vi "ATM front end.vi"() -> ()   [LabVIEW 2020]
uses:
  states_enum.ctl
  <vilib>/regexp/Match Regular Expression.xnode
panel:
  out "Card LED":bool
  in  "Right Button 3":bool
  in  "Right Button 2":bool
  in  "Right Button 1":bool
  in  "Left Button 3":bool
  in  "Left Button 2":bool
  in  "Left Button 1":bool
  out "Right 3":string
  out "Right 2":string
  out "Right 1":string
  out "Left 3":string
  out "Left 2":string
  out "Left 1":string
  out "Terminal":string
  in  "User Input":string
  in  "Enter":bool
  in  "Card Simulator":bool
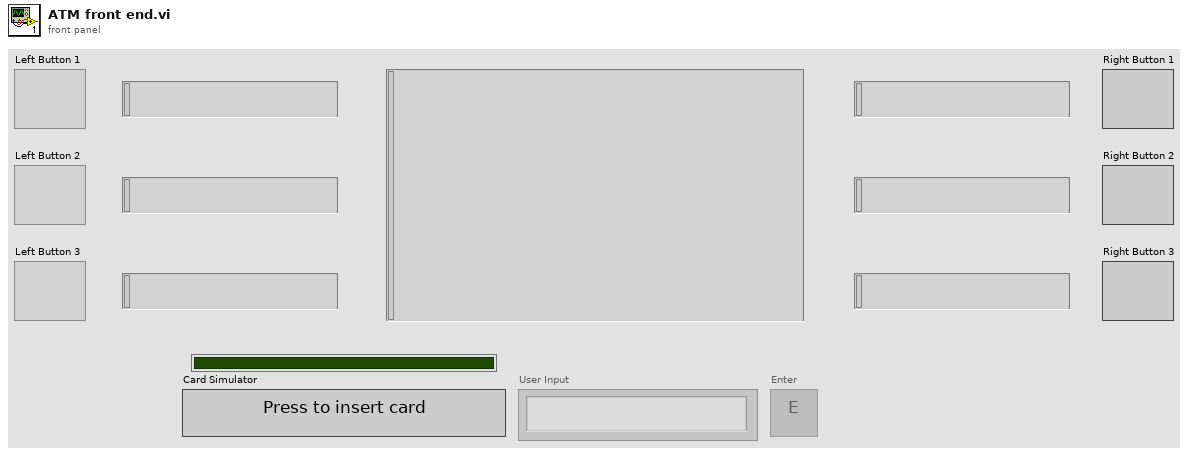
[diagram p1: front panel]
types:
  T1 = typedef "states_enum.ctl" = enum16{"Start", "Idle", "Validate card", "Enter account number", "Validate account", "Terminate session", "Main menu", "Balance Inquiry", "Deposit", "Fast Cash", "Withdraw", "Update account", "Transaction status"}
  T2 = enum8{"Enabled", "Disabled", "Disabled and Grayed Out"}
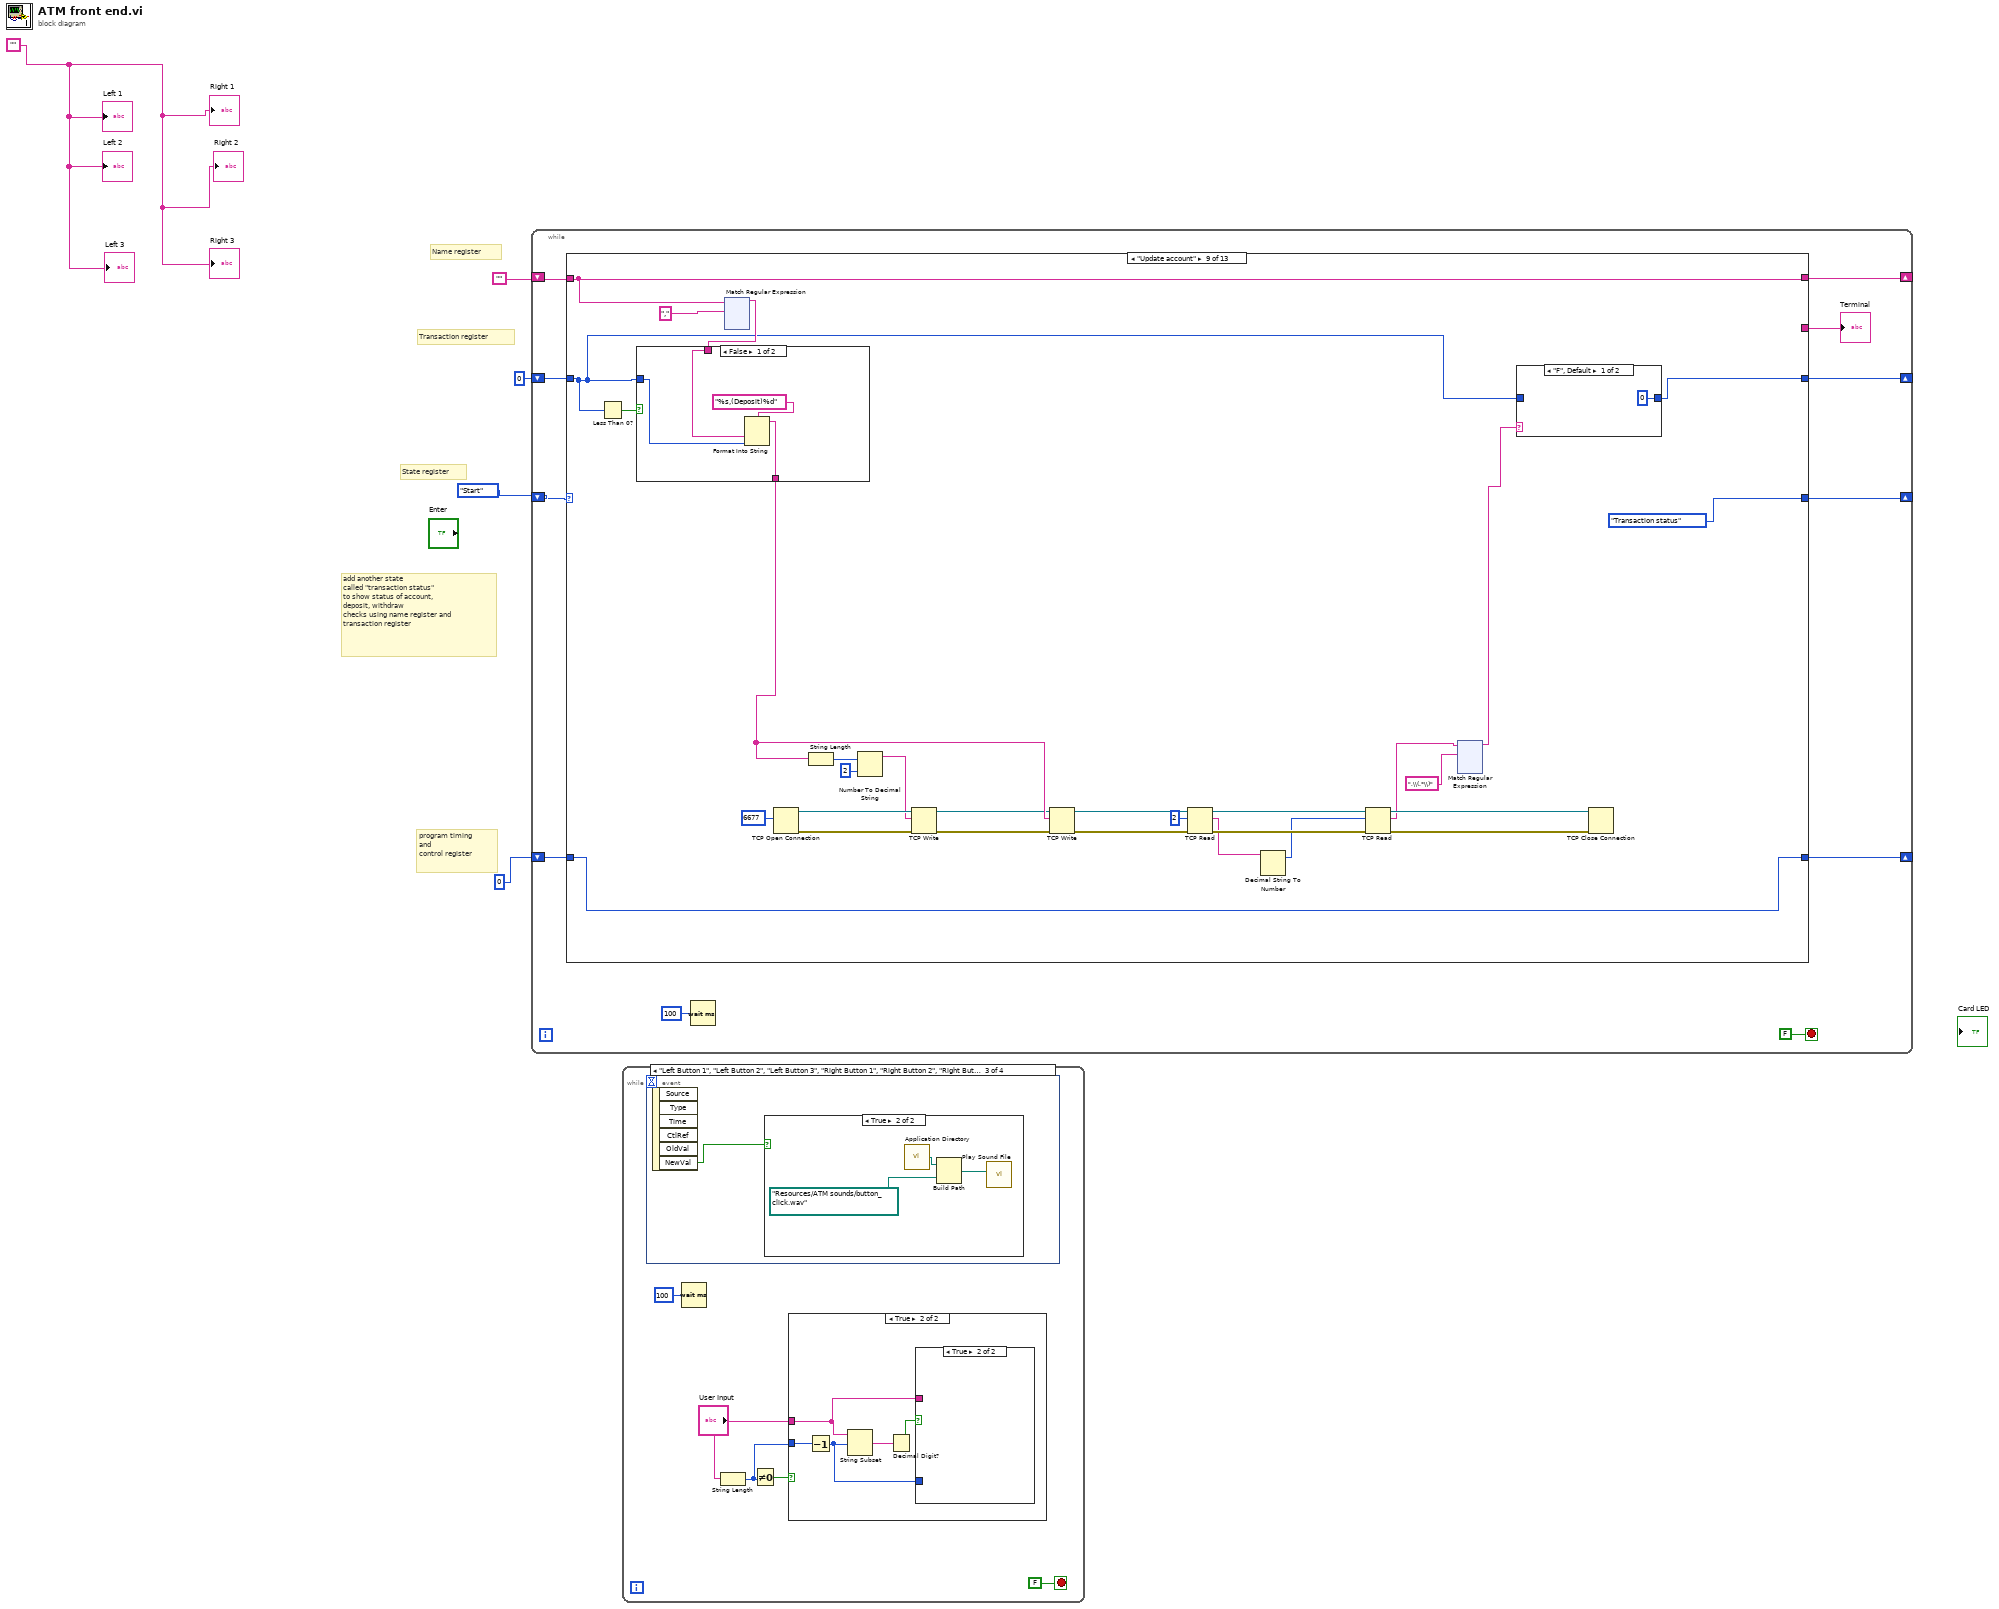
[diagram p0: block diagram]
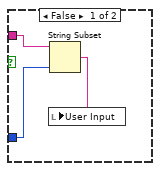
[diagram p3: hidden frame]
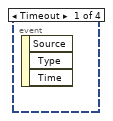
[diagram p4: hidden frame]
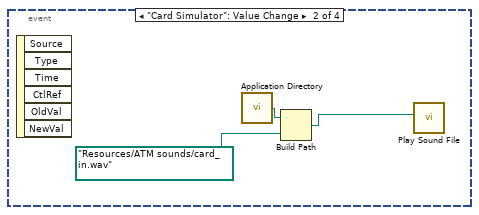
[diagram p5: hidden frame]
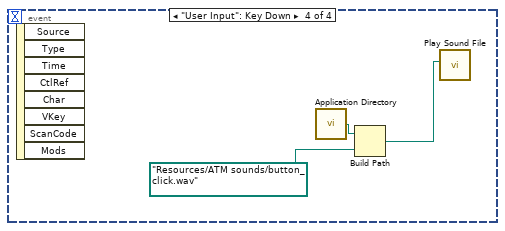
[diagram p7: hidden frame]
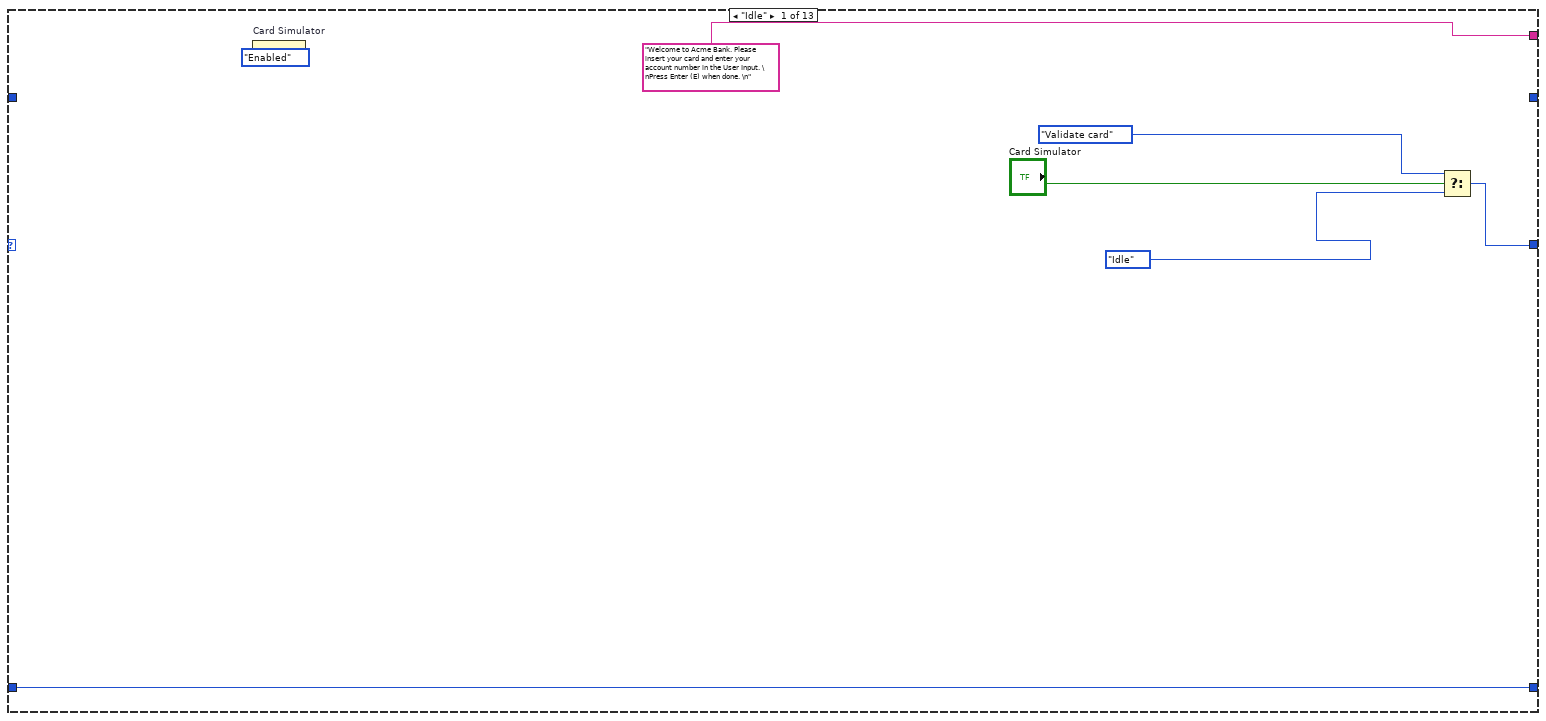
[diagram p8: hidden frame]
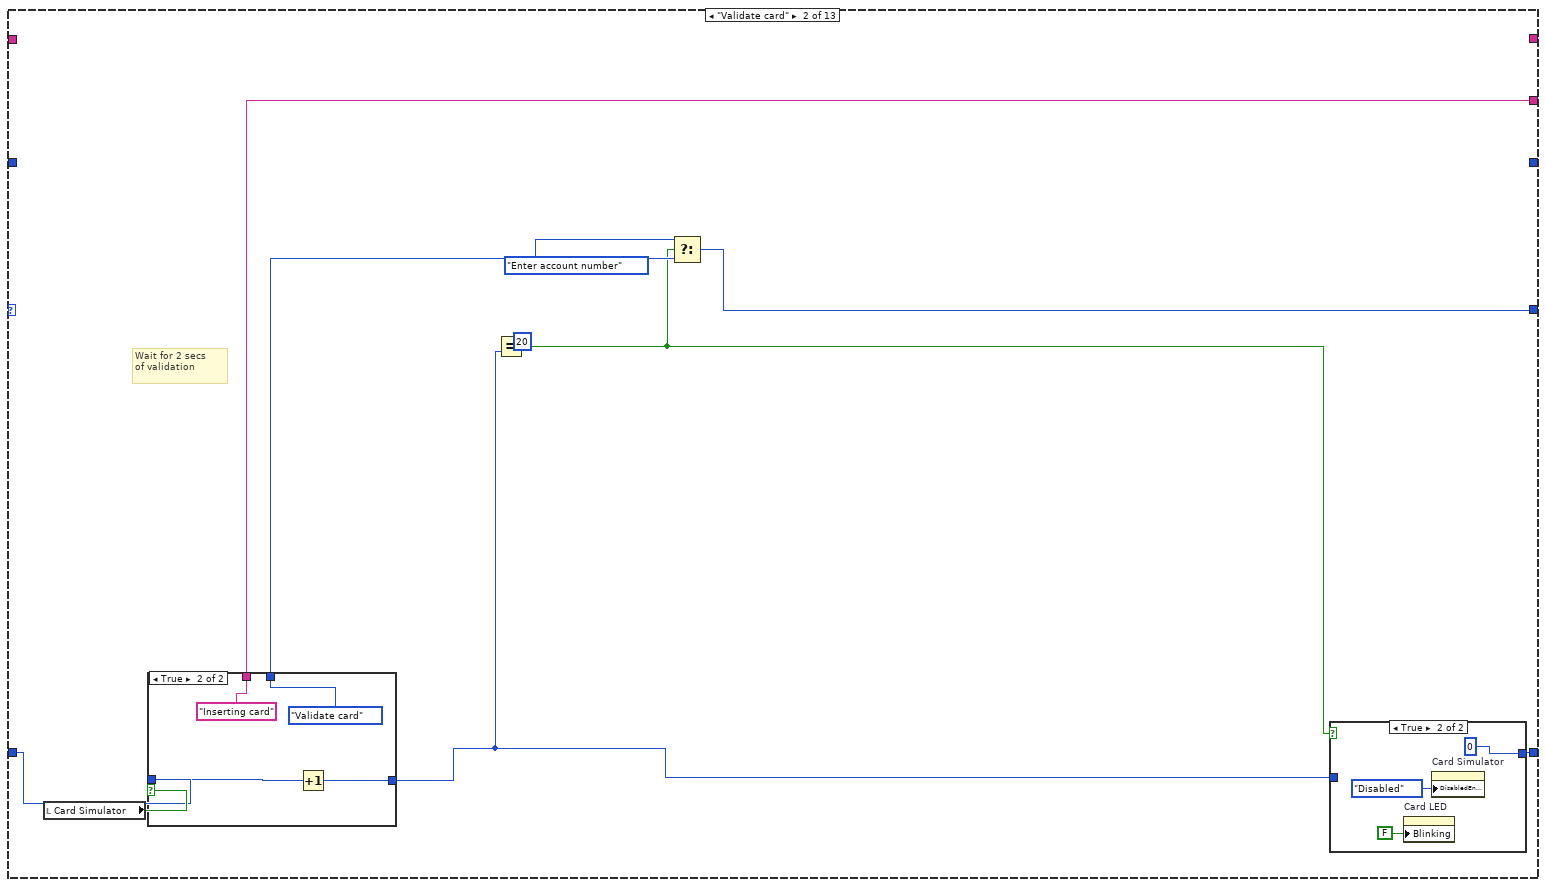
[diagram p9: hidden frame]
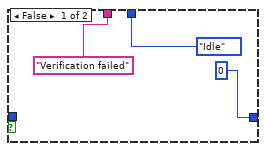
[diagram p10: hidden frame]
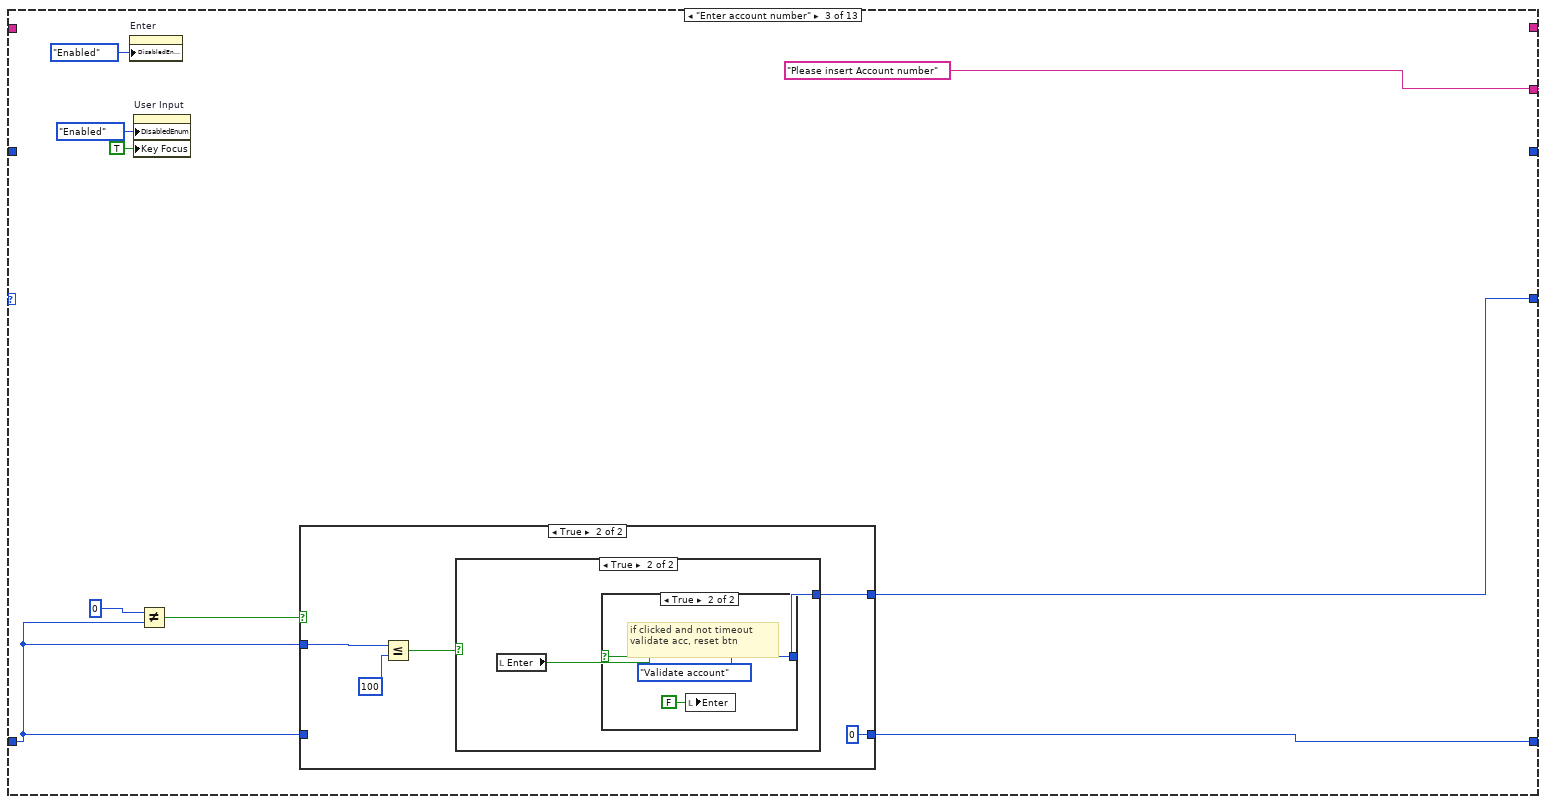
[diagram p12: hidden frame]
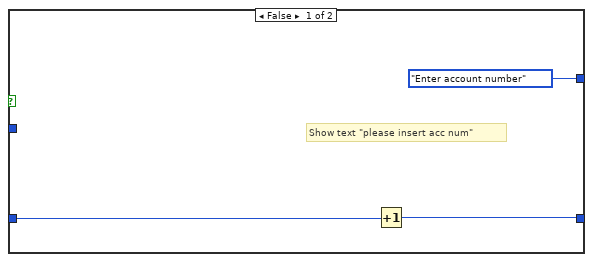
[diagram p13: hidden frame]
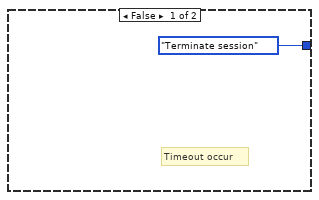
[diagram p14: hidden frame]
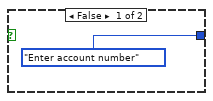
[diagram p15: hidden frame]
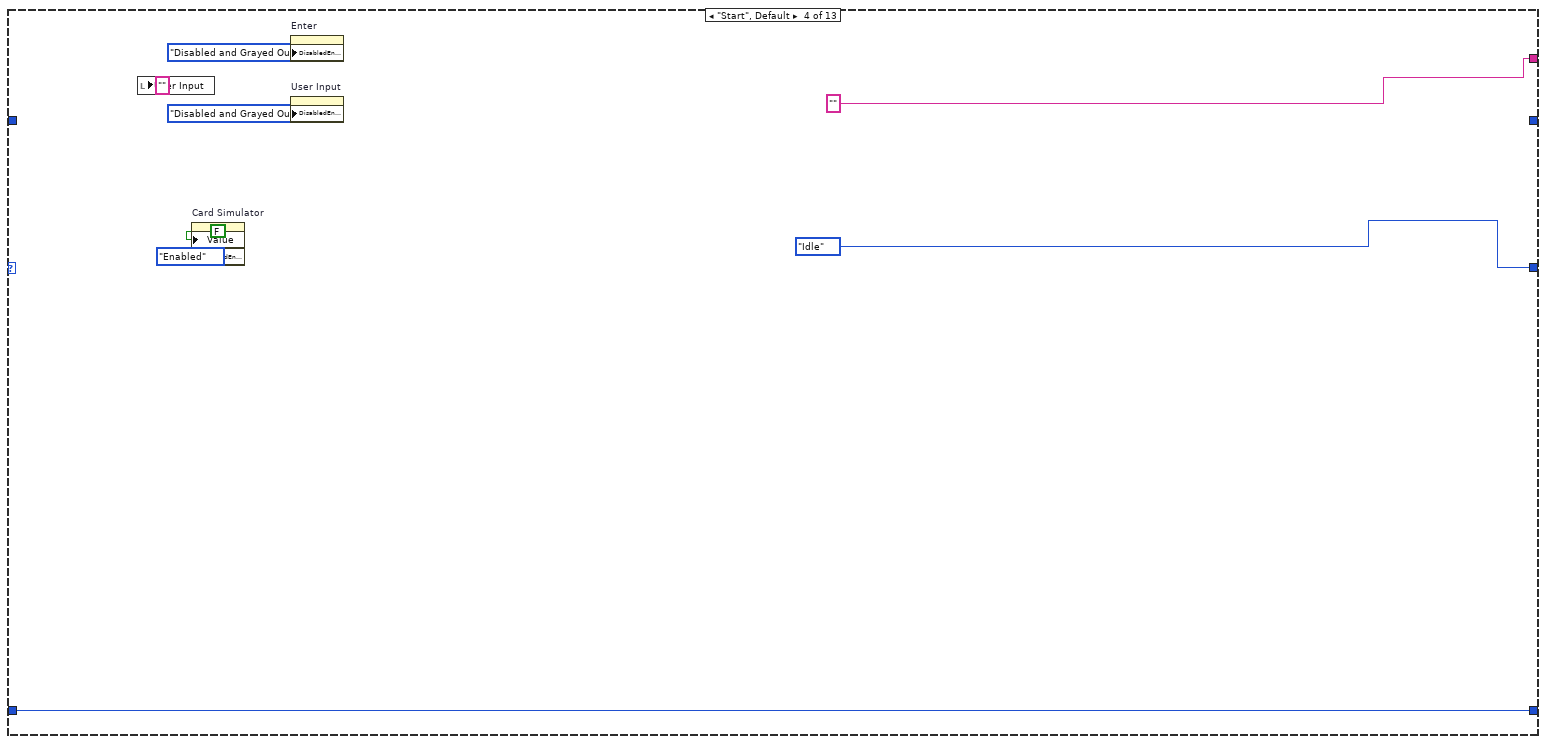
[diagram p16: hidden frame]
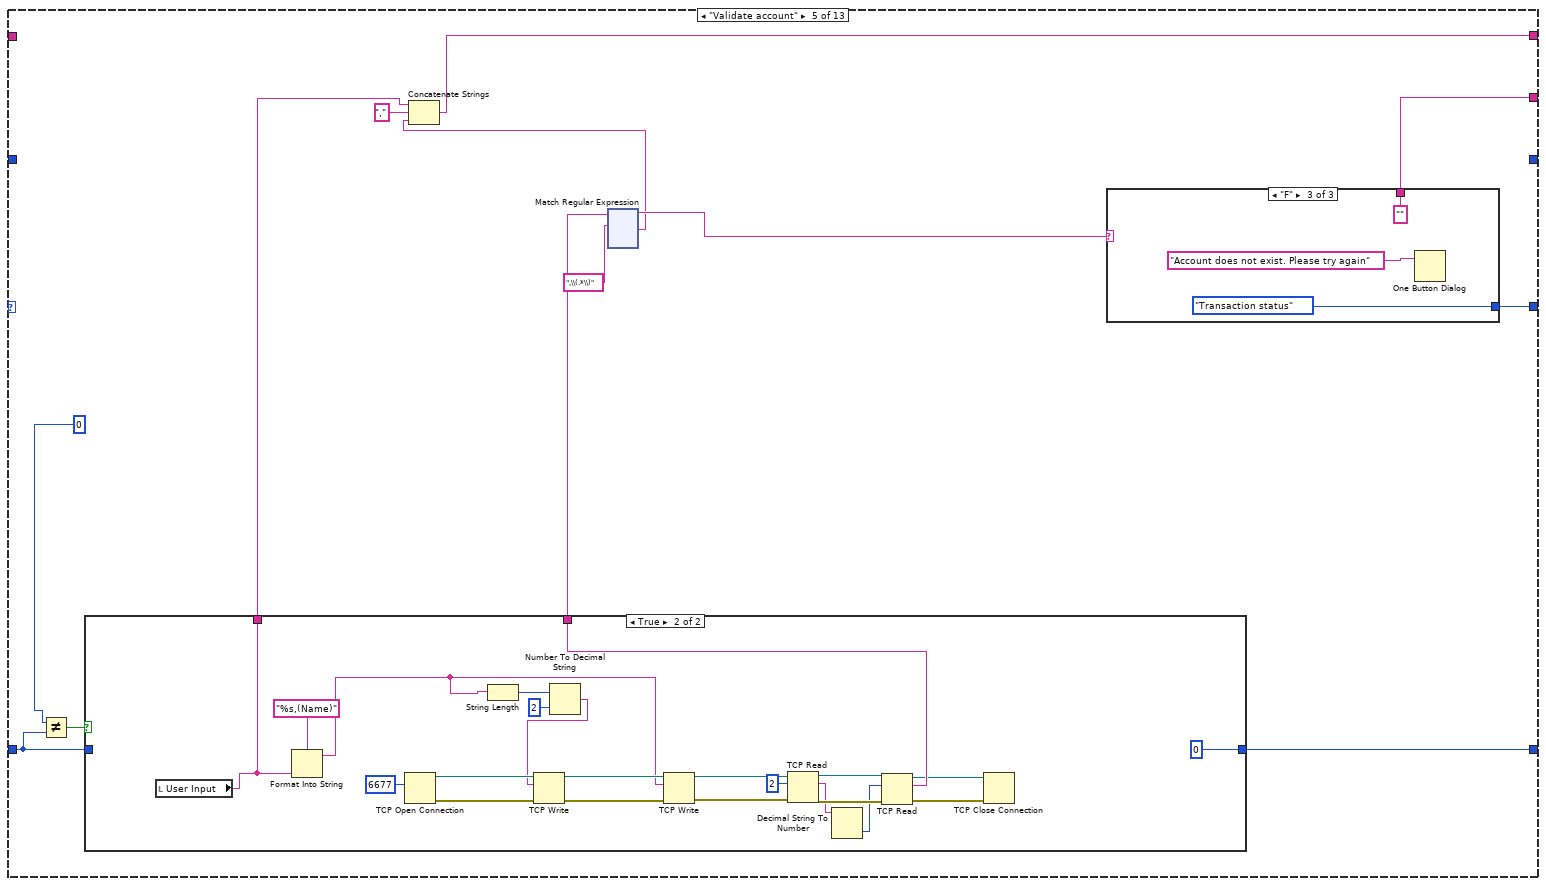
[diagram p17: hidden frame]
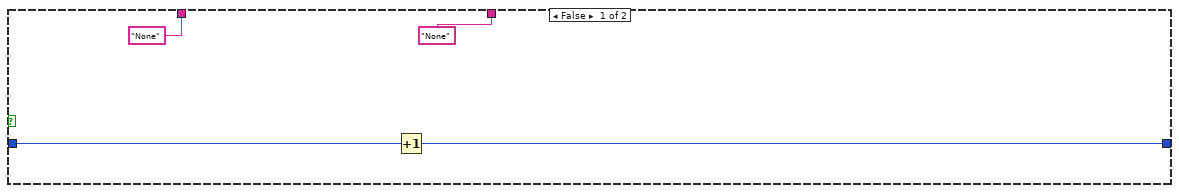
[diagram p18: hidden frame]
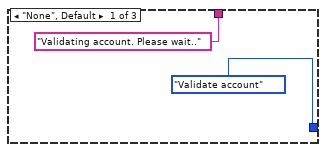
[diagram p19: hidden frame]
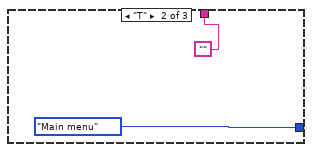
[diagram p20: hidden frame]
diagram:
  w4 = ""
  # "add another state\ncalled \"transaction status\"\nto show status of account, \ndeposit, withdraw\nchecks using name register and \ntransaction register"
  # "Transaction register"
  # "State register"
  # "program timing \nand \ncontrol register"
  # "Name register"
  n1 = while {
    shift-right: [w14] -> _
    shift-left: states_enum."Start" -> [w16]
    shift-right: [w11] -> _
    shift-left: 0 -> [w12]
    shift-right: [w8] -> _
    shift-left: "" -> [w9]
    shift-right: [w7] -> _
    shift-left: 0 -> [w6]
    stop <- FALSE stop-if-true
    n2 = case shown="\"Update account\"" w16 {
      tunnel: [w23 w32 w51 states_enum."Idle" w88 w241 w259 w436 states_enum."Transaction status" w975 w1013 states_enum."Update account" w1051] -> w14
      tunnel: ["Welcome to Acme Bank. Please insert your card and enter your account number in the User Input. \nPress Enter (E) when done. \n" ("Terminal") w27 "Please insert Account number" ("Terminal") "" ("Terminal") w76 "Your session has been terminated due to inactivity or menu selection. Please take your card \nGoodbye! \n" ("Terminal") w271 w437 _ "Please enter amount to deposit and press Enter (E) when done" ("Text.Text") "Please enter amount to withdraw and press Enter (E) when done" ("Text.Text") _ w1056] -> w13
      tunnel: w12 -> [w19 w29 w47 w74 w78 w246 w255 w439 w711 w977 w1014 w1046 w1054]
      tunnel: [w19 w24 w48 w74 w79 w242 w258 w438 w711 w976 w1011 w1046 w1055] -> w11
      tunnel: [_ _ _ _ w84 "" w266 w435 w710 w980 w1009 w1044 w1059] -> w8
      tunnel: w9 -> [_ _ _ _ _ _ w266 w435 w710 w980 w1009 w1044 w1059]
      tunnel: [_ _ _ _ _ _ _ _ w706 w974 w1010 -50 ("offset past number") w1049] -> w7
      tunnel: w6 -> [_ _ _ _ _ _ _ _ w707 _ _ _ w1050]
      frame "Idle" {
        n3 = property on="Card Simulator" class="Bool (strict)"("DisabledEnum"=T2."Enabled" ("Disabled")) -> ()  [unwired: 2 in, 2 out]
        n4 = Select(t=states_enum."Validate card", s="Card Simulator", f=states_enum."Idle") -> (s? t:f=w23:T1)
      }
      frame "Validate card" {
        # "Wait for 2 secs \nof validation"
        n5 = local read "Card Simulator"() -> (w30:bool)
        n6 = case shown="True" w30 {
          tunnel: w29 -> [_ w40]
          tunnel: [0 w39] -> w25
          tunnel: [states_enum."Idle" states_enum."Validate card"] -> w28
          tunnel: ["Verification failed" ("Terminal") "Inserting card" ("Terminal")] -> w27
          frame False {
          }
          frame True {
            n7 = Increment(x=w40) -> (x+1=w39:i32)
          }
        }
        n8 = Equal?(x=20, y=w25) -> (x = y?=w26:bool)
        n9 = Select(t=states_enum."Enter account number", s=w26, f=w28) -> (s? t:f=w32:T1)
        n10 = case shown="True" w26 {
          tunnel: w25 -> [w41 _]
          tunnel: [w41 0] -> w24
          frame False {
          }
          frame True {
            n11 = property on="Card LED" class="Bool (strict)"("Blinking"=FALSE) -> ()  [unwired: 2 in, 2 out]
            n12 = property on="Card Simulator" class="Bool (strict)"("DisabledEnum"=T2."Disabled" ("Disabled")) -> ()  [unwired: 2 in, 2 out]
          }
        }
      }
      frame "Enter account number" {
        n13 = property on="Enter" class="Bool (strict)"("DisabledEnum"=T2."Enabled" ("Disabled")) -> ()  [unwired: 2 in, 2 out]
        n14 = property on="User Input" class="Str"("DisabledEnum"=T2."Enabled" ("Disabled"), "Key Focus"=TRUE) -> ()  [unwired: 2 in, 2 out]
        n15 = Not Equal?(x=0, y=w47) -> (x != y?=w49:bool)
        n16 = case shown="True" w49 {
          tunnel: [states_enum."Enter account number" w57] -> w51
          tunnel: w47 -> [w56 _]
          tunnel: [w55 0] -> w48
          tunnel: w47 -> [_ w59]
          frame False {
            # "Show text \"please insert acc num\""
            n17 = Increment(x=w56) -> (x+1=w55:i32)
          }
          frame True {
            n18 = Less Or Equal?(x=w59, y=100) -> (x <= y?=w60:bool)
            n19 = case shown="True" w60 {
              tunnel: [states_enum."Terminate session" w63] -> w57
              frame False {
                # "Timeout occur"
              }
              frame True {
                n20 = local read "Enter"() -> (w64:bool)
                n21 = case shown="True" w64 {
                  tunnel: [states_enum."Enter account number" states_enum."Validate account"] -> w63
                  frame False {
                  }
                  frame True {
                    # "if clicked and not timeout\nvalidate acc, reset btn"
                    n22 = local write "Enter"(FALSE ("Enter")) -> ()
                  }
                }
              }
            }
          }
        }
      }
      frame "Start", Default {
        n23 = local write "User Input"("" ("User Input")) -> ()
        n24 = property on="Card Simulator" class="Bool (strict)"("Value"=FALSE ("Card Simulator"), "DisabledEnum"=T2."Enabled" ("Disabled")) -> ()  [unwired: 2 in, 2 out]
        n25 = property on="Enter" class="Bool (strict)"("DisabledEnum"=T2."Disabled and Grayed Out" ("Disabled")) -> ()  [unwired: 2 in, 2 out]
        n26 = property on="User Input" class="Str"("DisabledEnum"=T2."Disabled and Grayed Out" ("Disabled")) -> ()  [unwired: 2 in, 2 out]
      }
      frame "Validate account" {
        n27 = Not Equal?(x=0, y=w78) -> (x != y?=w81:bool)
        n28 = case shown="True" w81 {
          tunnel: ["None" ("data out") w114] -> w87
          tunnel: [w90 0] -> w79
          tunnel: w78 -> [w91 _]
          tunnel: ["None" ("User Input") w93] -> w77
          frame False {
            n29 = Increment(x=w91) -> (x+1=w90:i32)
          }
          frame True {
            n30 = local read "User Input"() -> (w93:string)
            n31 = Format Into String(format string="%s,(Name)", w93) -> (resulting string=w94:string)  [unwired: 2 in, 1 out]
            n32 = TCP Open Connection(remote port or service name=u16 6677) -> (connection ID=w113:refnum<k5>, error out=w111:errorcluster)  [unwired: 4 in]
            n33 = String Length(string=w94) -> (length=w107:i32)
            n34 = Number To Decimal String(number=w107, width (-)=i16 2) -> (decimal integer string=w108:string)
            n35 = TCP Write(connection ID=w113, data in=w108, error in (no error)=w111) -> (connection ID out=w112:refnum<k5>, error out=w110:errorcluster)  [unwired: 1 in, 1 out]
            n36 = TCP Write(connection ID=w112, data in=w94, error in (no error)=w110) -> (connection ID out=w105:refnum<k5>, error out=w100:errorcluster)  [unwired: 1 in, 1 out]
            n37 = TCP Read(connection ID=w105, bytes to read=2, error in (no error)=w100) -> (connection ID out=w104:refnum<k5>, data out=w98:string, error out=w101:errorcluster)  [unwired: 2 in]
            n38 = Decimal String To Number(string=w98) -> (number=w97:i32)  [unwired: 2 in, 1 out]
            n39 = TCP Read(connection ID=w104, bytes to read=w97, error in (no error)=w101) -> (connection ID out=w103:refnum<k5>, data out=w114:string, error out=w102:errorcluster)  [unwired: 2 in]
            n40 = TCP Close Connection(connection ID=w103, error in (no error)=w102) -> ()  [unwired: 1 in, 2 out]
          }
        }
        n41 = xnode "Match Regular Expression"("input string"=w87, "regular expression"=",\\(.*\\)") -> ("before match"=w86:string, "after match"=w82:string)  [unwired: 4 in, 3 out]
        n42 = Concatenate Strings(w77, "," ("string"), w82) -> (w84:string)
        n43 = case shown="\"F\"" w86 {
          tunnel: [states_enum."Validate account" states_enum."Main menu" states_enum."Transaction status"] -> w88
          tunnel: ["Validating account. Please wait.." ("Terminal") "" "" ("Terminal")] -> w76
          frame "None", Default {
          }
          frame "T" {
          }
          frame "F" {
            n44 = One Button Dialog(message="Account does not exist. Please try again" ("Terminal")) -> ()  [unwired: 1 in, 1 out]
          }
        }
      }
      frame "Terminate session" {
        w236 = ""
        n45 = local write "Right 1"(w236) -> ()
        n46 = local write "Left 2"(w236) -> ()
        n47 = local write "Right 2"(w236) -> ()
        n48 = local write "Left 3"(w236) -> ()
        n49 = local write "Left 1"(w236) -> ()
        n50 = local write "Right 3"(w236) -> ()
        n51 = local write "User Input"("" ("User Input")) -> ()
        n52 = property on="Card LED" class="Bool (strict)"("Blinking"=TRUE) -> ()  [unwired: 2 in, 2 out]
        n53 = property on="Card Simulator" class="Bool (strict)"("Value"=FALSE ("Card Simulator"), "DisabledEnum"=T2."Enabled" ("Disabled")) -> ()  [unwired: 2 in, 2 out]
        n54 = Increment(x=w246) -> (x+1=w243:i32)
        n55 = property on="Enter" class="Bool (strict)"("DisabledEnum"=T2."Disabled and Grayed Out" ("Disabled")) -> ()  [unwired: 2 in, 2 out]
        n56 = property on="User Input" class="Str"("DisabledEnum"=T2."Disabled and Grayed Out" ("Disabled")) -> ()  [unwired: 2 in, 2 out]
        n57 = Equal?(x=15, y=w243) -> (x = y?=w245:bool)
        n58 = case shown="False" w245 {
          tunnel: w243 -> [w252 _]
          tunnel: [w252 0] -> w242
          tunnel: [states_enum."Terminate session" states_enum."Idle"] -> w241
          frame False {
          }
          frame True {
          }
        }
      }
      frame "Main menu" {
        w269 = "\n"
        n59 = local write "User Input"("" ("User Input")) -> ()
        n60 = local write "Left 1"("None" ("Left 1")) -> ()
        n61 = local write "Left 2"("Balance Inquiry" ("Left 2")) -> ()
        n62 = local write "Left 3"("Return card and Terminate" ("Left 3")) -> ()
        n63 = local write "Right 1"("Deposit" ("Right 1")) -> ()
        n64 = local write "Right 2"("Withdraw" ("Right 2")) -> ()
        n65 = local write "Right 3"("Fast cash $50" ("Right 3")) -> ()
        n66 = xnode "Match Regular Expression"("input string"=w266, "regular expression"=",") -> ("after match"=w268:string)  [unwired: 4 in, 4 out]
        n67 = Not Equal To 0?(x=w255) -> (x != 0?=w257:bool)
        n68 = case shown="True" w257 {
          tunnel: [states_enum."Main menu" w278] -> w259
          tunnel: w255 -> [w275 w276]
          tunnel: [w274 w277] -> w258
          tunnel: w255 -> [_ w280]
          frame False {
            n69 = Increment(x=w275) -> (x+1=w274:i32)
          }
          frame True {
            n70 = Less Or Equal?(x=w280, y=100) -> (x <= y?=w281:bool)
            n71 = case shown="True" w281 {
              tunnel: [states_enum."Terminate session" w294] -> w278
              tunnel: [0 w292] -> w277
              tunnel: w276 -> [_ w293]
              frame False {
                # "Timeout occur"
              }
              frame True {
                # "0. None\n1. Balance\n2. Terminate\n3. Deposit\n4. Withdraw\n5. Fast cash"
                n72 = Build Array("Left Button 1", "Left Button 2", "Left Button 3", "Right Button 1", "Right Button 2", "Right Button 3") -> (w291:bool[])
                n73 = Search 1D Array(1D array=w291, element=TRUE) -> (index of element=w295:i32)  [unwired: 1 in]
                n74 = case shown="5" w295 {
                  tunnel: [states_enum."Main menu" states_enum."Main menu" states_enum."Balance Inquiry" states_enum."Terminate session" states_enum."Deposit" states_enum."Withdraw" states_enum."Fast Cash"] -> w294
                  tunnel: w293 -> [w297 _ _ _ _ _ _]
                  tunnel: [w296 0 0 0 0 0 0] -> w292
                  frame -1, Default {
                    n75 = Increment(x=w297) -> (x+1=w296:i32)
                  }
                  frame 0 {
                    # "No function,\nbut it breaks the\nprogram timeout"
                    n76 = local write "Left Button 1"(FALSE ("Left Button 2")) -> ()
                  }
                  frame 1 {
                    # "balance inquiry\nthen set the btn\nback to its original\nposition"
                    n77 = local write "Left Button 2"(FALSE ("Left Button 2")) -> ()
                  }
                  frame 2 {
                    n78 = local write "Left Button 3"(FALSE ("Left Button 2")) -> ()
                  }
                  frame 3 {
                    n79 = local write "Right Button 1"(FALSE ("Left Button 2")) -> ()
                  }
                  frame 4 {
                    n80 = local write "Right Button 2"(FALSE ("Left Button 2")) -> ()
                  }
                  frame 5 {
                    n81 = local write "Right Button 3"(FALSE ("Left Button 2")) -> ()
                  }
                }
              }
            }
          }
        }
        n82 = Concatenate Strings("Welcome to Acme Bank, ", w268, w269, w269, "Please select transaction by using the buttons") -> (w271:string)
      }
      frame "Balance Inquiry" {
        n83 = Equal To 0?(x=w439) -> (x = 0?=w440:bool)
        n84 = xnode "Match Regular Expression"("input string"=w435, "regular expression"=",") -> ("before match"=w431:string)  [unwired: 4 in, 4 out]
        n85 = Format Into String(format string="%s,(Balance)", w431) -> (resulting string=w433:string)  [unwired: 2 in, 1 out]
        n86 = case shown="False" w440 {
          tunnel: [w558 w587] -> w437
          tunnel: w439 -> [w557 w577]
          tunnel: [w556 w576] -> w438
          tunnel: [w555 states_enum."Balance Inquiry"] -> w436
          tunnel: w433 -> [_ w569]
          frame False {
            n87 = Less Or Equal?(x=w557, y=15) -> (x <= y?=w559:bool)
            n88 = case shown="True" w559 {
              tunnel: [0 w564] -> w556
              tunnel: w557 -> [_ w565]
              tunnel: [states_enum."Main menu" states_enum."Balance Inquiry"] -> w555
              frame False {
              }
              frame True {
                n89 = Increment(x=w565) -> (x+1=w564:i32)
              }
            }
            n90 = property on="Terminal" class="Str"() -> ("Text.Text"=w558:string)  [unwired: 2 in, 2 out]
          }
          frame True {
            n91 = TCP Open Connection(remote port or service name=u16 6677) -> (connection ID=w591:refnum<k5>, error out=w582:errorcluster)  [unwired: 4 in]
            n92 = String Length(string=w569) -> (length=w572:i32)
            n93 = Number To Decimal String(number=w572, width (-)=i16 2) -> (decimal integer string=w573:string)
            n94 = TCP Write(connection ID=w591, data in=w573, error in (no error)=w582) -> (connection ID out=w590:refnum<k5>, error out=w583:errorcluster)  [unwired: 1 in, 1 out]
            n95 = TCP Write(connection ID=w590, data in=w569, error in (no error)=w583) -> (connection ID out=w589:refnum<k5>, error out=w584:errorcluster)  [unwired: 1 in, 1 out]
            n96 = TCP Read(connection ID=w589, bytes to read=2, error in (no error)=w584) -> (connection ID out=w588:refnum<k5>, data out=w579:string, error out=w585:errorcluster)  [unwired: 2 in]
            n97 = Decimal String To Number(string=w579) -> (number=w578:i32)  [unwired: 2 in, 1 out]
            n98 = TCP Read(connection ID=w588, bytes to read=w578, error in (no error)=w585) -> (connection ID out=w581:refnum<k5>, data out=w568:string, error out=w580:errorcluster)  [unwired: 2 in]
            n99 = Increment(x=w577) -> (x+1=w576:i32)
            n100 = xnode "Match Regular Expression"("input string"=w568, "regular expression"="\\(.*\\)") -> ("after match"=w566:string)  [unwired: 4 in, 4 out]
            n101 = Format Into String(format string="Your balance is :\\n $%s", w566) -> (resulting string=w587:string)  [unwired: 2 in, 1 out]
            n102 = TCP Close Connection(connection ID=w581, error in (no error)=w580) -> ()  [unwired: 1 in, 2 out]
          }
        }
      }
      frame "Update account" {
        n103 = Less Than 0?(x=w707) -> (x < 0?=w733:bool)
        n104 = xnode "Match Regular Expression"("input string"=w710, "regular expression"=",") -> ("before match"=w732:string)  [unwired: 4 in, 4 out]
        n105 = case shown="False" w733 {
          tunnel: w732 -> [w736 w742]
          tunnel: [w737 w743] -> w731
          tunnel: w707 -> [w735 w740]
          frame False {
            n106 = Format Into String(format string="%s,(Deposit)%d", w736, w735) -> (resulting string=w737:string)  [unwired: 2 in, 1 out]
          }
          frame True {
            n107 = Negate(x=w740) -> (-x=w739:i32)
            n108 = Format Into String(format string="%s,(Withdraw)%d", w742, w739) -> (resulting string=w743:string)  [unwired: 2 in, 1 out]
          }
        }
        n109 = TCP Open Connection(remote port or service name=u16 6677) -> (connection ID=w729:refnum<k5>, error out=w720:errorcluster)  [unwired: 4 in]
        n110 = String Length(string=w731) -> (length=w718:i32)
        n111 = Number To Decimal String(number=w718, width (-)=i16 2) -> (decimal integer string=w717:string)
        n112 = TCP Write(connection ID=w729, data in=w717, error in (no error)=w720) -> (connection ID out=w728:refnum<k5>, error out=w721:errorcluster)  [unwired: 1 in, 1 out]
        n113 = TCP Write(connection ID=w728, data in=w731, error in (no error)=w721) -> (connection ID out=w727:refnum<k5>, error out=w722:errorcluster)  [unwired: 1 in, 1 out]
        n114 = TCP Read(connection ID=w727, bytes to read=2, error in (no error)=w722) -> (connection ID out=w726:refnum<k5>, data out=w716:string, error out=w723:errorcluster)  [unwired: 2 in]
        n115 = Decimal String To Number(string=w716) -> (offset past number=w715:i32)  [unwired: 2 in, 1 out]
        n116 = TCP Read(connection ID=w726, bytes to read=w715, error in (no error)=w723) -> (connection ID out=w725:refnum<k5>, data out=w712:string, error out=w724:errorcluster)  [unwired: 2 in]
        n117 = xnode "Match Regular Expression"("input string"=w712, "regular expression"=",\\(.*\\)") -> ("before match"=w730:string)  [unwired: 4 in, 4 out]
        n118 = case shown="\"F\", Default" w730 {
          tunnel: w707 -> [_ w973]
          tunnel: [0 w973] -> w706
          frame "F", Default {
          }
          frame "T" {
          }
        }
        n119 = TCP Close Connection(connection ID=w725, error in (no error)=w724) -> ()  [unwired: 1 in, 2 out]
      }
      frame "Deposit" {
        n120 = Not Equal To 0?(x=w977) -> (x != 0?=w978:bool)
        n121 = property on="User Input" class="Str"("Key Focus"=TRUE) -> ()  [unwired: 2 in, 2 out]
        n122 = case shown="True" w978 {
          tunnel: w977 -> [w985 w987]
          tunnel: [w984 w988] -> w976
          tunnel: [states_enum."Deposit" w989] -> w975
          tunnel: [0 w986] -> w974
          frame False {
            # "no transaction yet"
            # "display the \"please enter\" text"
            n123 = Increment(x=w985) -> (x+1=w984:i32)
          }
          frame True {
            n124 = Less Or Equal?(x=w987, y=100) -> (x <= y?=w990:bool)
            n125 = case shown="True" w990 {
              tunnel: [states_enum."Terminate session" w999] -> w989
              tunnel: [0 w995] -> w988
              tunnel: w987 -> [_ w998]
              tunnel: [0 w997] -> w986
              frame False {
                # "reset transaction amnt"
                # "Timeout occur"
              }
              frame True {
                n126 = Increment(x=w998) -> (x+1=w996:i32)
                n127 = local read "Enter"() -> (w1000:bool)
                n128 = case shown="True" w1000 {
                  tunnel: [states_enum."Deposit" states_enum."Update account"] -> w999
                  tunnel: [0 w1005] -> w997
                  tunnel: [w1001 0] -> w995
                  tunnel: w996 -> [w1001 _]
                  frame False {
                    # "no transaction yet"
                  }
                  frame True {
                    # "reset counter"
                    # "send transaction\namnt to next state"
                    # "reset btn position"
                    # "If clicked, proceed to update acc"
                    n129 = local write "Enter"(FALSE ("Enter")) -> ()
                    n130 = local read "User Input"() -> (w1006:string)
                    n131 = Decimal String To Number(string=w1006) -> (number=w1005:i32)  [unwired: 2 in, 1 out]
                  }
                }
              }
            }
          }
        }
      }
      frame "Withdraw" {
        n132 = Not Equal To 0?(x=w1014) -> (x != 0?=w1015:bool)
        n133 = case shown="True" w1015 {
          tunnel: [w1020 w1023] -> w1011
          tunnel: [states_enum."Withdraw" w1024] -> w1013
          tunnel: [0 w1022] -> w1012
          tunnel: w1014 -> [w1017 w1021]
          frame False {
            # "no transaction yet"
            # "display the \"please enter\" text"
            n134 = Increment(x=w1017) -> (x+1=w1020:i32)
          }
          frame True {
            n135 = Less Or Equal?(x=w1021, y=100) -> (x <= y?=w1025:bool)
            n136 = case shown="True" w1025 {
              tunnel: [states_enum."Terminate session" w1034] -> w1024
              tunnel: [0 w1030] -> w1023
              tunnel: [0 w1033] -> w1022
              tunnel: w1021 -> [_ w1032]
              frame False {
                # "reset transaction amnt"
                # "Timeout occur"
              }
              frame True {
                n137 = Increment(x=w1032) -> (x+1=w1031:i32)
                n138 = local read "Enter"() -> (w1035:bool)
                n139 = case shown="True" w1035 {
                  tunnel: [states_enum."Withdraw" states_enum."Update account"] -> w1034
                  tunnel: [0 w1040] -> w1033
                  tunnel: w1031 -> [w1036 _]
                  tunnel: [w1036 0] -> w1030
                  frame False {
                    # "no transaction yet"
                  }
                  frame True {
                    # "reset \ncounter"
                    # "send transaction\namnt to next state"
                    # "reset btn position"
                    # "If clicked, proceed to update acc"
                    n140 = local write "Enter"(FALSE ("Enter")) -> ()
                    n141 = local read "User Input"() -> (w1041:string)
                    n142 = Decimal String To Number(string=w1041) -> (number=w1040:i32)  [unwired: 2 in, 1 out]
                  }
                }
              }
            }
          }
        }
        n143 = Negate(x=w1012) -> (-x=w1010:i32)
      }
      frame "Fast Cash" {
      }
      frame "Transaction status" {
        n144 = xnode "Match Regular Expression"("input string"=w1059, "regular expression"=",") -> ("after match"=w1057:string)  [unwired: 4 in, 4 out]
        n145 = Empty String/Path?(string/path=w1057) -> (empty?=w1048:bool)
        n146 = case shown="False" w1048 {
          tunnel: w1050 -> [w1067 _]
          tunnel: [w1068 "Account Information Incorrect Please Re-Enter Account Number. \nPress Enter (E) when done "] -> w1056
          frame False {
            n147 = Equal To 0?(x=w1067) -> (x = 0?=w1069:bool)
            n148 = case shown="False" w1069 {
              tunnel: [w1074 "Insufficient funds in account Please check your balance and try again "] -> w1068
              tunnel: w1067 -> [w1071 _]
              frame False {
                n149 = Greater Than 0?(x=w1071) -> (x > 0?=w1073:bool)
                n150 = Negate(x=w1071) -> (-x=w1072:i32)
                n151 = Select(t="$%d Deposited", s=w1073, f="$%d Withdrawn") -> (s? t:f=w1075:string)
                n152 = Select(t=w1071, s=w1073, f=w1072) -> (s? t:f=w1070:i32)
                n153 = Format Into String(format string=w1075, w1070) -> (resulting string=w1074:string)  [unwired: 2 in, 1 out]
              }
              frame True {
                # "If withdrawal failed"
              }
            }
          }
          frame True {
          }
        }
        n154 = Less?(x=w1054, y=20) -> (x < y?=w1052:bool)
        n155 = case shown="False" w1052 {
          tunnel: [w1062 states_enum."Transaction status"] -> w1051
          tunnel: w1050 -> [_ w1065]
          tunnel: [0 w1065] -> w1049
          tunnel: w1048 -> [w1060 _]
          frame False {
            n156 = Select(t=states_enum."Enter account number", s=w1060, f=states_enum."Main menu") -> (s? t:f=w1062:T1)
          }
          frame True {
          }
        }
        n157 = Increment(x=w1054) -> (x+1=w1055:i32)
      }
    }
    "Terminal" <- w13
    n158 = Wait (ms)(milliseconds to wait=u32 100) -> ()  [unwired: 1 out]
  }
  n159 = while {
    stop <- FALSE stop-if-true
    n160 = event shown="[2] \"Left Button 1\", \"Left Button 2\", \"Left Button 3\", \"Right Button 1\", \"Right Button 2\", \"Right Button 3\", \"Enter\": Value Change" {
      selector: _ -> [_ _ _ _]
      dyn-events: _ -> [_ _ _ _]
      timeout: _ -> [_ _ _ _]
      event Timeout {
        n161 = event-data() -> ()  [unwired: 1 in, 3 out]
      }
      event "Card Simulator": Value Change {
        n162 = event-data() -> ()  [unwired: 1 in, 6 out]
        n163 = call <vilib>:"Application Directory.vi"() -> ("Application Directory"=w1209:path)
        n164 = Build Path(base path=w1209, name or relative path=path "Resources/ATM sounds/card_in.wav" ("file path (dialog if empty)")) -> (appended path=w1207:path)
        n165 = call <vilib>:"Play Sound File.vi"("path"=w1207) -> ()  [unwired: 9 in, 2 out]
      }
      event "Left Button 1", "Left Button 2", "Left Button 3", "Right Button 1", "Right Button 2", "Right Button 3", "Enter": Value Change {
        n166 = event-data() -> ("NewVal"=w1210:bool)  [unwired: 1 in, 5 out]
        n167 = case shown="True" w1210 {
          frame False {
          }
          frame True {
            n168 = call <vilib>:"Application Directory.vi"() -> ("Application Directory"=w1213:path)
            n169 = Build Path(base path=w1213, name or relative path=path "Resources/ATM sounds/button_click.wav" ("file path (dialog if empty)")) -> (appended path=w1211:path)
            n170 = call <vilib>:"Play Sound File.vi"("path"=w1211) -> ()  [unwired: 9 in, 2 out]
          }
        }
      }
      event "User Input": Key Down {
        n171 = event-data() -> ()  [unwired: 1 in, 8 out]
        n172 = call <vilib>:"Application Directory.vi"() -> ("Application Directory"=w1216:path)
        n173 = Build Path(base path=w1216, name or relative path=path "Resources/ATM sounds/button_click.wav" ("file path (dialog if empty)")) -> (appended path=w1214:path)
        n174 = call <vilib>:"Play Sound File.vi"("path"=w1214) -> ()  [unwired: 9 in, 2 out]
      }
    }
    n175 = Wait (ms)(milliseconds to wait=u32 100) -> ()  [unwired: 1 out]
    n176 = String Length(string="User Input") -> (length=w1196:i32)
    n177 = Not Equal To 0?(x=w1196) -> (x != 0?=w1194:bool)
    n178 = case shown="True" w1194 {
      tunnel: "User Input" -> [_ w1200]
      tunnel: w1196 -> [_ w1203]
      frame False {
      }
      frame True {
        n179 = Decrement(x=w1203) -> (x-1=w1199:i32)
        n180 = String Subset(string=w1200, offset (0)=w1199) -> (substring=w1202:string)  [unwired: 1 in]
        n181 = Decimal Digit?(1:w1202) -> (0:w1201:bool)
        n182 = case shown="True" w1201 {
          tunnel: w1200 -> [w1206 _]
          tunnel: w1199 -> [w1205 _]
          frame False {
            n183 = String Subset(string=w1206, length (rest)=w1205) -> (substring=w1204:string)  [unwired: 1 in]
            n184 = local write "User Input"(w1204) -> ()
          }
          frame True {
          }
        }
      }
    }
  }
  "Left 1" <- w4
  "Left 2" <- w4
  "Left 3" <- w4
  "Right 1" <- w4
  "Right 2" <- w4
  "Right 3" <- w4
